vi "Task Stop.vi"(8 "error in (no error)":errorcluster, 11 "SimTask in":refnum<class "SimTask.lvclass">) -> (0 "error out":errorcluster, 3 "SimTask out":refnum<class "SimTask.lvclass">)   [LabVIEW 2020, in "VolatusDemo.lvlib" / "SimTask.lvclass"]
uses:
  SimTask.lvclass
  SimTask.lvclass/SimTask.ctl
  Volatus/Task/Task.lvclass
  C:/dev/lv20CE/relink/lv-volatus/Volatus/Task/Task.lvclass
  C:/Program Files (x86)/National Instruments/LabVIEW 2020/vi.lib/ActorFramework/Actor/Actor.lvclass
  C:/dev/lv20CE/relink/lv-volatus/Volatus/APIRegistrationHandler/APIRegistrationHandler.lvclass
  C:/dev/lv20CE/relink/lv-volatus/Volatus/TaskStateHandler/TaskStateHandler.lvclass
  C:/dev/lv20CE/relink/lv-volatus/Volatus/VectoMessageHandler/VectoMessageHandler.lvclass
  C:/dev/lv20CE/relink/lv-volatus/VolatusDemo/SimTask/SimTask.lvclass
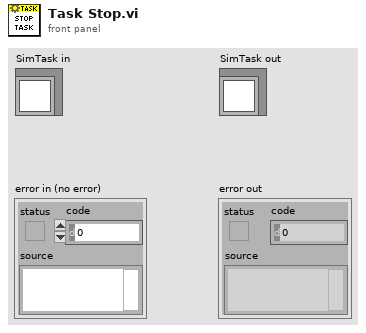
[diagram p1: front panel]
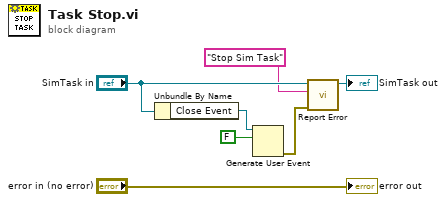
[diagram p0: block diagram]
diagram:
  n1 = Unbundle By Name("SimTask in") -> ("Close Event"=w5:refnum<user-event>)
  n2 = Generate User Event(user event=w5, event data cluster=FALSE ("event data")) -> (error out=w1:errorcluster)  [unwired: 2 in, 1 out]
  n3 = call "Report Error.vi"("error in (no error)"=w1, "Context"="Stop Sim Task", "Task in"="SimTask in") -> ("Task out"=→"SimTask out":refnum<class "SimTask.lvclass">)  [unwired: 7 in, 1 out]
  "error out" <- "error in (no error)"
